vi "Image roto-translation top level.vi"(0 "ROI to crop (pixels)":T7={"Xmax"=2147483647, "Ymax"=2147483647, "Xmin"=0, "Ymin"=0}, 1 "Theta range (deg)":T6={"theta max (deg)"=180.0, "theta min (deg)"=-180.0}, 2 "Txy range (pixels)":T3={"Tx max (pix)"=2147483647, "Tx min (pix)"=-2147483648, "Ty max (pix)"=2147483647, "Ty min (pix)"=-2147483648}, 3 "Convergence tolerances":T4={"Tx,y tol (abs pix)"=0.001, "Rotation tol (abs deg)"=0.001, "Scale tol (rel fact)"=0.001}, 4 "Max. iters":i32=20, 5 "Controls":T2={"Auto ROI (for rot.)"=FALSE, "Apply scaling"=FALSE, "Apply rotation"=TRUE, "Apply Tx"=TRUE, "Apply Ty"=TRUE, "Keep proc. img"=FALSE}, 6 "Test image file path":path, 7 "R_min":dbl=150.0, 8 "Reference image file path":path, 9 "Pre-scale iters":i32=2) -> (12 "Iter":i32, 13 "Converged":bool, 14 "Scale factor":dbl, 15 "Rotation (deg)":dbl, 16 "Tx (pixels)":dbl, 17 "Ty (pixels)":dbl, 18 "Processed test img path":path, 19 "Error Out":errorcluster)   [LabVIEW 2022 SP3]
uses:
  Typedefs/ROI bounds.ctl
  Typedefs/Theta range.ctl
  Typedefs/Txy range.ctl
  Typedefs/Top level controls.ctl
  <vilib>/vision/NI_Vision_Development_Module.lvlib
panel:
  in  "ROI Color":u32(colorbox)=16711935
  out "Test image overlayed onto reference image (blend)":T1(plugin-control)
  out "Test image transformed":T1(plugin-control)
  out "Test image":T1(plugin-control)
  out "Convergence":T5(graph)
  out "Reference image":T1(plugin-control)
  # "ROI and Txy (pixels) are in image array coordinates. Origin is at top left, so positive y is towards the bottom of the image. positive x is towards the right of the image."
  # "Reference image info"
  # "Transformations are of test image relative to reference image, in image array coordinates"
  # "Paul Nathan 10/06/2015, \n07/12/2015, 22/03/2016, 06/04/2016, 19/04/2016, 23/06/2016"
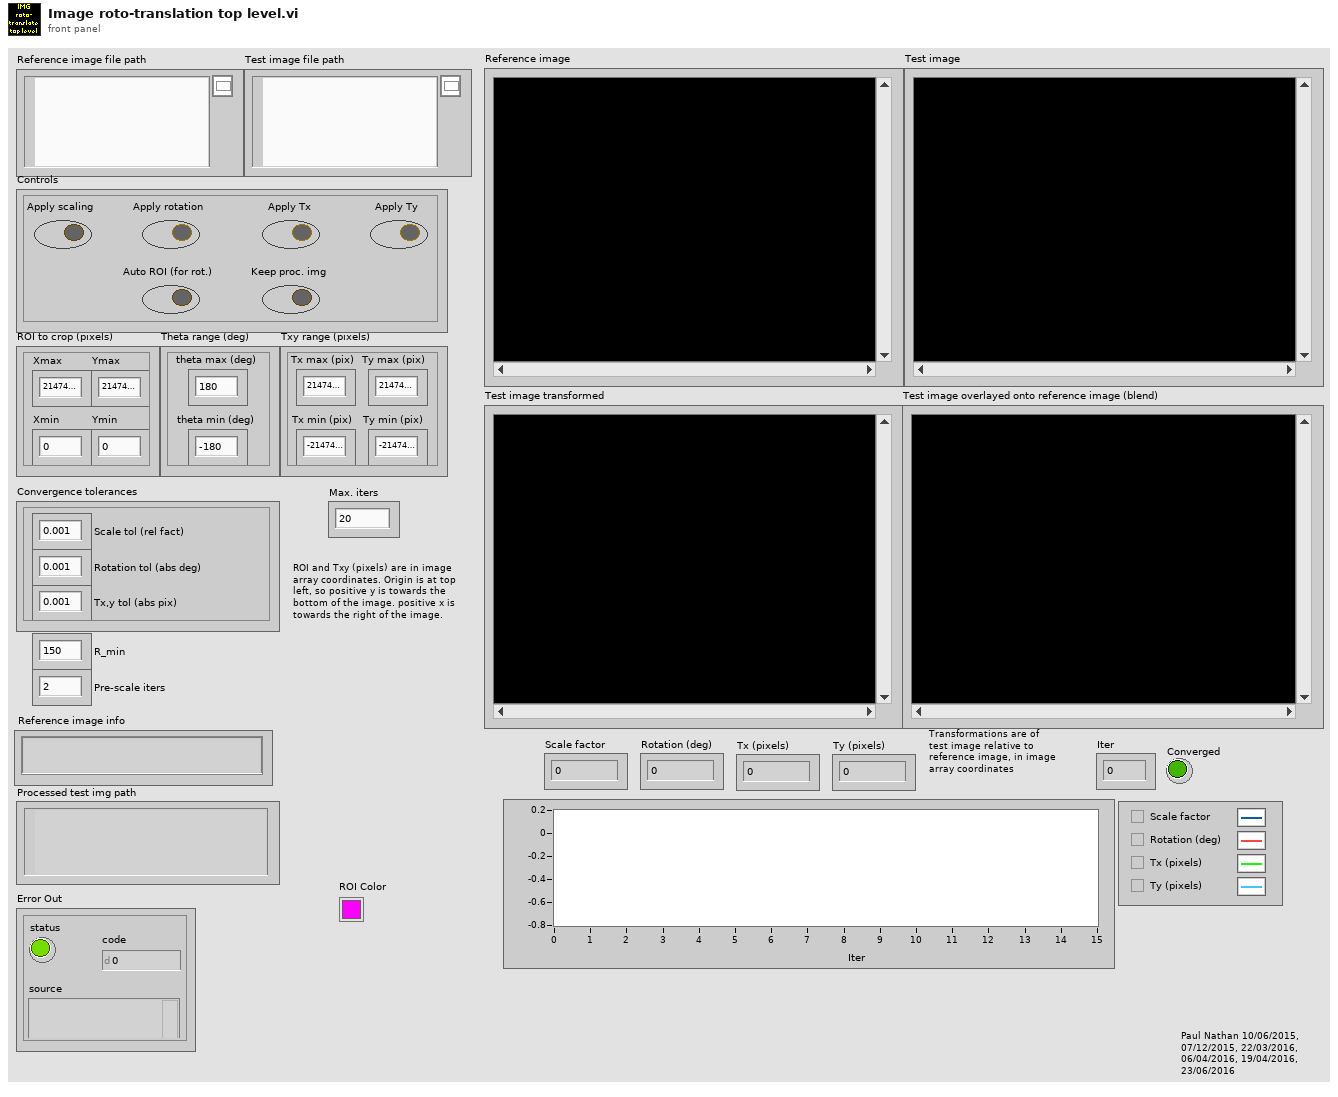
[diagram p1: front panel]
types:
  T1 = typedef "IMAQ Image.ctl" = refnum<image>
  T2 = typedef "Top level controls.ctl" = cluster{"Auto ROI (for rot.)":bool, "Apply scaling":bool, "Apply rotation":bool, "Apply Tx":bool, "Apply Ty":bool, "Keep proc. img":bool}
  T3 = typedef "Txy range.ctl" = cluster{"Tx max (pix)":i32, "Tx min (pix)":i32, "Ty max (pix)":i32, "Ty min (pix)":i32}
  T4 = cluster{"Tx,y tol (abs pix)":dbl, "Rotation tol (abs deg)":dbl, "Scale tol (rel fact)":dbl}
  T5 = cluster{dbl, dbl, "dx (pix)":dbl, "dy (pix)":dbl}
  T6 = typedef "Theta range.ctl" = cluster{"theta max (deg)":dbl, "theta min (deg)":dbl}
  T7 = typedef "ROI bounds.ctl" = cluster{"Xmax":i32, "Ymax":i32, "Xmin":i32, "Ymin":i32}
  T8 = cluster{dbl, dbl, "dx (pix)":dbl, "dy (pix)":dbl}[]
  T9 = typedef "Image Type" = u32
  T10 = cluster{"Xmin":i32, "Ymin":i32, "Xmax":i32, "Ymax":i32}
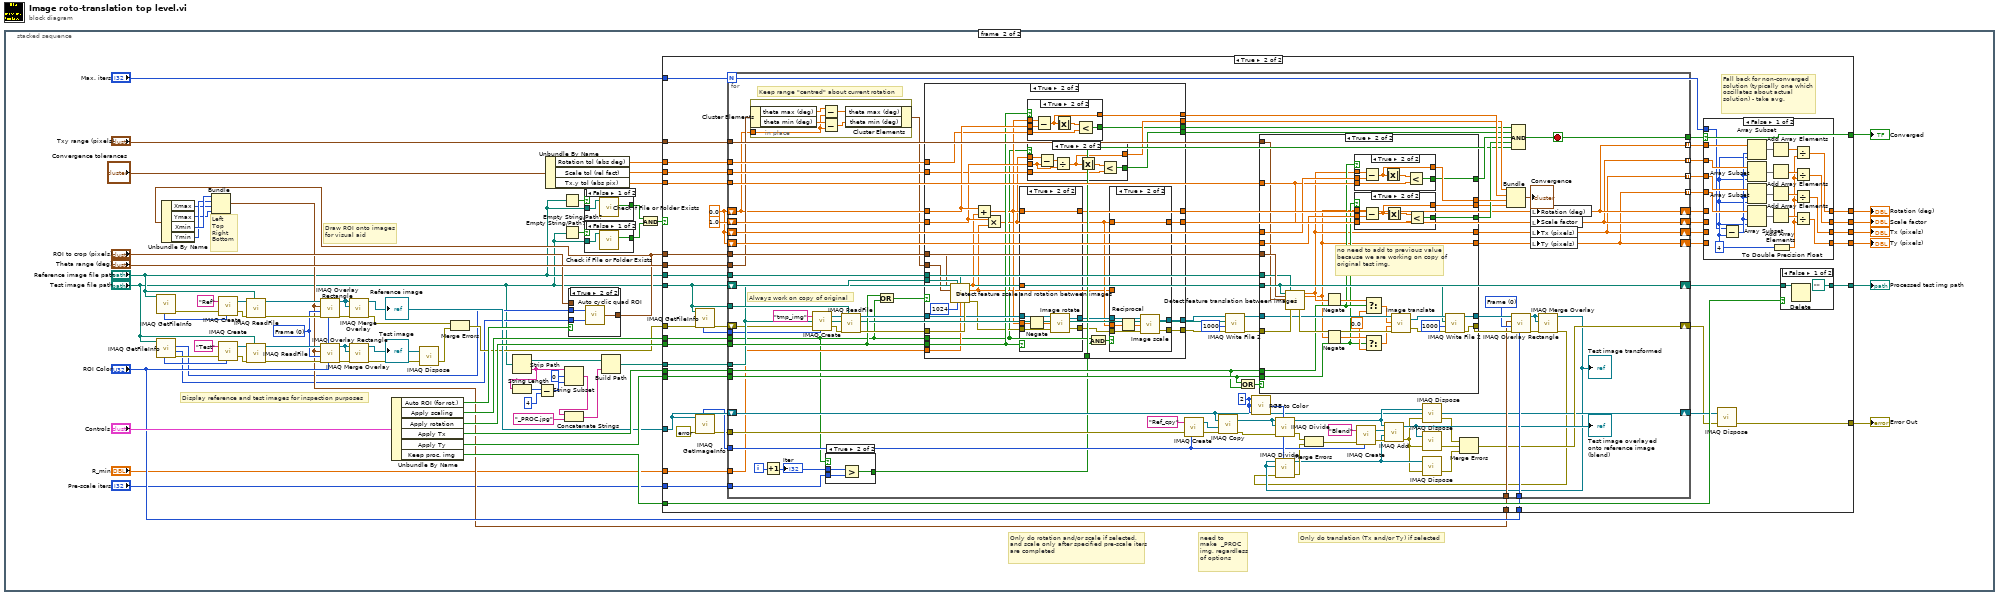
[diagram p0: block diagram]
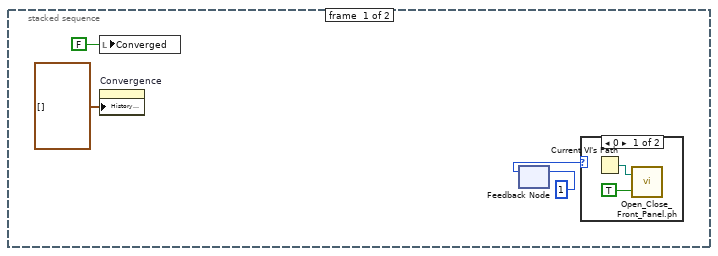
[diagram p2: hidden frame]
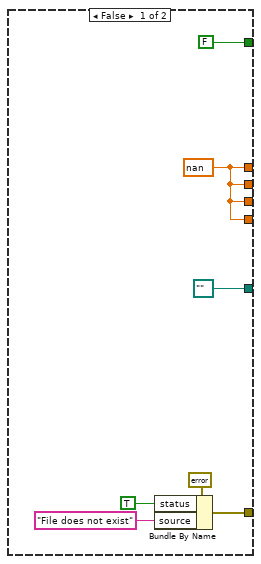
[diagram p4: hidden frame]
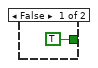
[diagram p5: hidden frame]
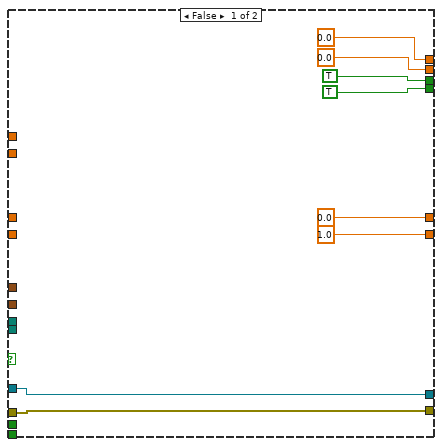
[diagram p6: hidden frame]
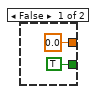
[diagram p7: hidden frame]
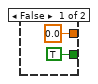
[diagram p8: hidden frame]
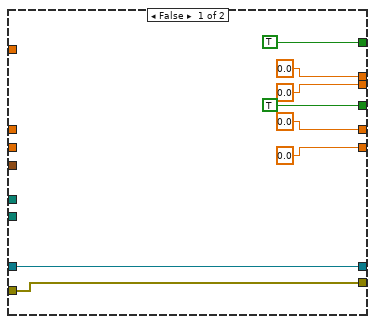
[diagram p11: hidden frame]
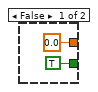
[diagram p12: hidden frame]
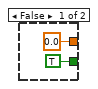
[diagram p13: hidden frame]
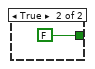
[diagram p16: hidden frame]
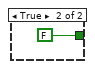
[diagram p17: hidden frame]
diagram:
  n1 = stacked-sequence {
    frame #0 {
      n2 = local write "Converged"(FALSE ("Converged")) -> ()
      n3 = property on="Convergence" class="WFChart (strict)"("History Data"=T8 []) -> ()  [unwired: 2 in, 2 out]
      n4 = feedback #1() -> (w2:i32)  [unwired: 1 in]
      n5 = feedback-in #1(1) -> ()
      n6 = case shown="0" w2 {
        frame 0 {
          n7 = Current VI's Path() -> (path=w5:path)
          n8 = call "Open_Close_Front_Panel.ph.vi"("openWindow (T)"=TRUE ("Front Panel Window:Open"), "VI path"=w5) -> ()  [unwired: 1 in, 1 out]
        }
        frame Default {
        }
      }
    }
    frame #1 {
      w29 = u32 0 items=["Frame", "Fill", "Highlight"] ("Drawing Mode (Frame)")
      # "Draw ROI onto images for visual aid"
      # "Display reference and test images for inspection purposes"
      # "Left\nTop\nRight\nBottom"
      # "Only do translation (Tx and/or Ty) if selected"
      # "Only do rotation and/or scale if selected,\nand scale only after specified pre-scale iters are completed"
      # "need to make  _PROC img, regardless of options"
      n9 = call "IMAQ GetFileInfo"("File Path"="Reference image file path") -> ("error out"=w45:errorcluster, "Image Type"=w44:T9)  [unwired: 4 in, 5 out]
      n10 = call "IMAQ GetFileInfo"("File Path"="Test image file path") -> ("error out"=w42:errorcluster, "Y Resolution"=w17:i32, "X Resolution"=w18:i32, "Image Type"=w43:T9)  [unwired: 4 in, 3 out]
      n11 = call "IMAQ Create"("Image Name"="Ref", "Image Type"=w44, "error in (no error)"=w45) -> ("New Image"=w47:T1, "error out"=w46:errorcluster)  [unwired: 2 in]
      n12 = call "IMAQ Create"("Image Name"="Test", "Image Type"=w43, "error in (no error)"=w42) -> ("New Image"=w40:T1, "error out"=w41:errorcluster)  [unwired: 2 in]
      n13 = call "IMAQ ReadFile"("File Path"="Reference image file path", "error in (no error)"=w46, "Image"=w47) -> ("error out"=w37:errorcluster, "Image Out"=w38:T1)  [unwired: 4 in, 3 out]
      n14 = call "IMAQ ReadFile"("File Path"="Test image file path", "error in (no error)"=w41, "Image"=w40) -> ("error out"=w30:errorcluster, "Image Out"=w31:T1)  [unwired: 4 in, 3 out]
      n15 = Unbundle By Name("Controls") -> ("Auto ROI (for rot.)"=w52:bool, "Apply scaling"=w51:bool, "Apply rotation"=w53:bool, "Apply Tx"=w54:bool, "Apply Ty"=w55:bool, "Keep proc. img"=w56:bool)
      n16 = Strip Path(path="Test image file path") -> (stripped path=w73:path, name=w79:string)
      n17 = String Length(string=w79) -> (length=w78:i32)
      n18 = Subtract(x=w78, y=4) -> (x-y=w72:i32)
      n19 = Unbundle By Name("Convergence tolerances") -> ("Rotation tol (abs deg)"=w60:dbl, "Scale tol (rel fact)"=w59:dbl, "Tx,y tol (abs pix)"=w58:dbl)
      n20 = Empty String/Path?(string/path="Reference image file path") -> (empty?=w10:bool)
      n21 = Empty String/Path?(string/path="Test image file path") -> (empty?=w8:bool)
      n22 = String Subset(string=w79, offset (0)=0, length (rest)=w72) -> (substring=w76:string)
      n23 = Concatenate Strings(w76, "_PROC.jpg" ("name or relative path")) -> (w74:string)
      n24 = case shown="True" w52 {
        tunnel: [w390 w391] -> w11
        tunnel: w18 -> [_ w393]
        tunnel: w17 -> [_ w392]
        tunnel: "ROI to crop (pixels)" -> [w390 _]
        frame False {
        }
        frame True {
          n25 = call "Auto cyclic quad ROI.vi"("img_H"=w392, "img_W"=w393) -> ("ROI to crop (pixels)"=w391:T7)
        }
      }
      n26 = Unbundle By Name(w11) -> ("Xmax"=w33:i32, "Ymax"=w32:i32, "Xmin"=w35:i32, "Ymin"=w34:i32)
      n27 = Bundle("Xmin"=w35, "Ymin"=w34, "Xmax"=w33, "Ymax"=w32) -> (w27:T10)  [unwired: 1 in]
      n28 = call "IMAQ Overlay Rectangle"("Color"="ROI Color", "error in (no error)"=w37, "Drawing Mode (Frame)"=w29, "Rectangle"=w27, "Image"=w38) -> ("error out"=w25:errorcluster, "Image Out"=w16:T1)  [unwired: 5 in]
      n29 = call "IMAQ Overlay Rectangle"("Color"="ROI Color", "error in (no error)"=w30, "Drawing Mode (Frame)"=w29, "Rectangle"=w27, "Image"=w31) -> ("error out"=w21:errorcluster, "Image Out"=w15:T1)  [unwired: 5 in]
      n30 = call "IMAQ Merge Overlay"("error in (no error)"=w25, "Image Dst"=w16, "Image Src"=w16) -> ("error out"=w24:errorcluster, "Image Dst Out"=w23:T1)  [unwired: 7 in]
      "Reference image" <- w23
      n31 = call "IMAQ Merge Overlay"("error in (no error)"=w21, "Image Dst"=w15, "Image Src"=w15) -> ("error out"=w20:errorcluster, "Image Dst Out"=w22:T1)  [unwired: 7 in]
      "Test image" <- w22
      n32 = call "IMAQ Dispose"("Image"=w22, "error in (no error)"=w20) -> ("error out"=w26:errorcluster)  [unwired: 4 in]
      n33 = Merge Errors(w24, w26) -> (w19:errorcluster)
      n34 = case shown="False" w10 {
        tunnel: [w388 FALSE ("file or folder exists?")] -> w67
        tunnel: "Reference image file path" -> [w387 _]
        frame False {
          n35 = call <vilib>:"Check if File or Folder Exists.vi"("path"=w387) -> ("file or folder exists?"=w388:bool)  [unwired: 8 in, 2 out]
        }
        frame True {
        }
      }
      n36 = case shown="False" w8 {
        tunnel: [w385 FALSE ("file or folder exists?")] -> w68
        tunnel: "Test image file path" -> [w384 _]
        frame False {
          n37 = call <vilib>:"Check if File or Folder Exists.vi"("path"=w384) -> ("file or folder exists?"=w385:bool)  [unwired: 8 in, 2 out]
        }
        frame True {
        }
      }
      n38 = Build Path(base path=w73, name or relative path=w74) -> (appended path=w80:path)
      n39 = And(x=w67, y=w68) -> (x .and. y?=w66:bool)
      n40 = case shown="True" w66 {
        tunnel: "Reference image file path" -> [_ w101]
        tunnel: "Max. iters" -> [_ w89]
        tunnel: w80 -> [_ w134]
        tunnel: [w86 w114] -> w63
        tunnel: [w86 w110] -> w64
        tunnel: "Test image file path" -> [_ w105]
        tunnel: [w86 w112] -> w62
        tunnel: w51 -> [_ w133]
        tunnel: w53 -> [_ w132]
        tunnel: w11 -> [_ w131]
        tunnel: w54 -> [_ w130]
        tunnel: w55 -> [_ w129]
        tunnel: "Theta range (deg)" -> [_ w128]
        tunnel: [path "" ("Test image file path") w125] -> w69
        tunnel: [w84 w96] -> w65
        tunnel: w56 -> [_ w127]
        tunnel: [w86 w108] -> w14
        tunnel: w60 -> [_ w122]
        tunnel: w59 -> [_ w121]
        tunnel: w58 -> [_ w120]
        tunnel: "Txy range (pixels)" -> [_ w119]
        tunnel: [FALSE w106] -> w49
        tunnel: w23 -> [_ w95]
        tunnel: w19 -> [_ w104]
        tunnel: "ROI Color" -> [_ w100]
        tunnel: w27 -> [_ w99]
        tunnel: "R_min" -> [_ w91]
        tunnel: "Pre-scale iters" -> [_ w90]
        frame False {
          w86 = nan ("Rotation (deg)")
          n41 = Bundle By Name(cluster=errorcluster {"status"=FALSE, "code"=0, "source"=""} ("error in (no error)"), "status"=TRUE, "source"="File does not exist") -> (w84:errorcluster)
        }
        frame True {
          w123 = 0.0 ("Rotation (deg)")
          # "Fall back for non-converged solution (typically one which oscillates about actual solution) - take avg."
          n42 = call "IMAQ GetImageInfo"("error in (no error)"=errorcluster {"status"=FALSE, "code"=0, "source"=""}, "Image"=w95) -> ("error out"=w92:errorcluster, "Image Type"=w94:T9)  [unwired: 2 in, 6 out]
          n43 = call "IMAQ GetFileInfo"("error in (no error)"=w104, "File Path"=w105) -> ("error out"=w103:errorcluster, "Image Type"=w102:T9)  [unwired: 3 in, 5 out]
          n44 = for {
            N: w89 -> [_]
            tunnel: w101 -> [w194]
            shift-right: [w190] -> w126
            shift-left: w105 -> [w219]
            tunnel: w134 -> [w190]
            shift-right: [w148] -> w97
            shift-left: w103 -> [w177]
            tunnel: w133 -> [w135]
            tunnel: w132 -> [w195]
            tunnel: w131 -> [w218]
            tunnel: w130 -> [w192]
            tunnel: w129 -> [w193]
            tunnel: w128 -> [w184]
            tunnel: w105 -> [w212]
            shift-right: [w181] -> w113
            shift-left: w123 -> [w183]
            shift-right: [w180] -> w111
            shift-left: 1.0 ("Rotation (deg)") -> [w205]
            shift-right: [w179] -> w109
            shift-left: w123 -> [w203]
            shift-right: [w142] -> w107
            shift-left: w123 -> [w202]
            tunnel: w122 -> [w208]
            tunnel: w121 -> [w197]
            tunnel: w120 -> [w196]
            tunnel: w119 -> [w185]
            tunnel: [w181] -> w118 mode=indexing
            tunnel: [w180] -> w117 mode=indexing
            tunnel: [w179] -> w116 mode=indexing
            tunnel: [w142] -> w115 mode=indexing
            tunnel: [w178] -> w106
            tunnel: w102 -> [w176]
            tunnel: w92 -> [w161]
            tunnel: w94 -> [w163]
            tunnel: w100 -> [w171]
            tunnel: w99 -> [w170]
            shift-right: [w147] -> w98
            shift-left: w95 -> [w147]
            tunnel: w91 -> [w140]
            tunnel: w90 -> [w137]
            i -> [w139]
            stop <- w178 stop-if-true
            w169 = u8 2 ("R")
            w172 = u32 0 items=["Frame", "Fill", "Highlight"] ("Drawing Mode (Frame)")
            # "Keep range \"centred\" about current rotation"
            # "Always work on copy of original"
            n45 = in-place {
              in-place-border: w183 -> [w226]
              n46 = in-place-cluster #2(w184) -> ("theta max (deg)"=w228:dbl, "theta min (deg)"=w227:dbl)
              n47 = Subtract(x=w228, y=w226) -> (x-y=w225:dbl)
              n48 = Subtract(x=w227, y=w226) -> (x-y=w224:dbl)
              n49 = in-place-cluster #2("theta max (deg)"=w225, "theta min (deg)"=w224) -> (w182:T6)
            }
            n50 = Increment(x=w139) -> (x+1=w138:i32)
            "Iter" <- w138
            n51 = call "IMAQ Create"("Image Name"="tmp_img", "Image Type"=w176, "error in (no error)"=w177) -> ("New Image"=w216:T1, "error out"=w217:errorcluster)  [unwired: 2 in]
            n52 = case shown="True" w135 {
              tunnel: w138 -> [_ w223]
              tunnel: w137 -> [_ w222]
              tunnel: [TRUE w221] -> w136
              frame False {
              }
              frame True {
                n53 = Greater?(x=w223, y=w222) -> (0:w221:bool)
              }
            }
            n54 = call "IMAQ ReadFile"("File Path"=w212, "error in (no error)"=w217, "Image"=w216) -> ("error out"=w214:errorcluster, "Image Out"=w213:T1)  [unwired: 4 in, 3 out]
            n55 = Or(x=w195, y=w135) -> (x .or. y?=w186:bool)
            n56 = case shown="True" w186 {
              tunnel: w219 -> [_ w267]
              tunnel: w218 -> [_ w266]
              tunnel: w182 -> [_ w265]
              tunnel: w214 -> [w229 w264]
              tunnel: w213 -> [w230 w263]
              tunnel: w183 -> [_ w262]
              tunnel: w208 -> [_ w261]
              tunnel: [0.0 w260] -> w207
              tunnel: [0.0 w259] -> w206
              tunnel: w205 -> [_ w258]
              tunnel: [TRUE w257] -> w201
              tunnel: [TRUE w256] -> w200
              tunnel: w197 -> [_ w255]
              tunnel: [1.0 w243] -> w180
              tunnel: [0.0 w246] -> w181
              tunnel: w135 -> [_ w240]
              tunnel: w195 -> [_ w254]
              tunnel: w194 -> [_ w253]
              tunnel: [w229 w249] -> w188
              tunnel: [w230 w248] -> w187
              tunnel: w140 -> [_ w241]
              tunnel: w136 -> [_ w238]
              frame False {
              }
              frame True {
                n57 = call "Detect feature scale and rotation between images.vi"("ROI to crop (pixels)"=w266, "Test image file path"=w267, "Reference image file path"=w253, "Theta range (deg)"=w265, "Log-polar transform size"=1024, "R_min"=w241, "Error In"=w264) -> ("Rotation (deg)"=w245:dbl, "Scale factor"=w242:dbl, "Error out"=w252:errorcluster)  [unwired: 4 in, 2 out]
                n58 = Add(x=w262, y=w245) -> (x+y=w247:dbl)
                n59 = Multiply(x=w258, y=w242) -> (x*y=w244:dbl)
                n60 = case shown="True" w254 {
                  tunnel: w263 -> [w287 w290]
                  tunnel: w252 -> [w286 w294]
                  tunnel: w247 -> [_ w291]
                  tunnel: [w287 w293] -> w251
                  tunnel: [w286 w292] -> w250
                  tunnel: w247 -> [_ w288]
                  tunnel: [w285 w288] -> w246
                  tunnel: w245 -> [w285 _]
                  frame False {
                  }
                  frame True {
                    n61 = Negate(x=w291) -> (-x=w289:dbl)
                    n62 = call "Image rotate.vi"("Error in"=w294, "Rotation angle, ccw+ (deg)"=w289, "Image in"=w290) -> ("Error Out"=w292:errorcluster, "Image Out"=w293:T1)
                  }
                }
                n63 = case shown="True" w254 {
                  tunnel: w262 -> [_ w284]
                  tunnel: w261 -> [_ w283]
                  tunnel: [0.0 w281] -> w260
                  tunnel: [TRUE w280] -> w257
                  tunnel: w247 -> [_ w279]
                  frame False {
                  }
                  frame True {
                    n64 = Subtract(x=w279, y=w284) -> (x-y=w281:dbl)
                    n65 = Absolute Value(x=w281) -> (abs(x)=w282:dbl)
                    n66 = Less?(x=w282, y=w283) -> (x < y?=w280:bool)
                  }
                }
                n67 = case shown="True" w240 {
                  tunnel: [0.0 w275] -> w259
                  tunnel: w258 -> [_ w273]
                  tunnel: [TRUE w272] -> w256
                  tunnel: w255 -> [_ w271]
                  tunnel: w244 -> [_ w270]
                  frame False {
                  }
                  frame True {
                    n68 = Subtract(x=w270, y=w273) -> (x-y=w276:dbl)
                    n69 = Divide(x=w276, y=w273) -> (x/y=w275:dbl)
                    n70 = Absolute Value(x=w275) -> (abs(x)=w274:dbl)
                    n71 = Less?(x=w274, y=w271) -> (x < y?=w272:bool)
                  }
                }
                n72 = And(x=w240, y=w238) -> (x .and. y?=w239:bool)
                n73 = case shown="True" w239 {
                  tunnel: w251 -> [w297 w304]
                  tunnel: [w297 w303] -> w248
                  tunnel: w250 -> [w296 w302]
                  tunnel: [w296 w301] -> w249
                  tunnel: w244 -> [_ w300]
                  tunnel: w244 -> [_ w298]
                  tunnel: [w295 w298] -> w243
                  tunnel: w242 -> [w295 _]
                  frame False {
                  }
                  frame True {
                    n74 = Reciprocal(x=w300) -> (1/x=w299:dbl)
                    n75 = call "Image scale.vi"("Error in"=w302, "Scale factor"=w299, "Image in"=w304) -> ("Error Out"=w301:errorcluster, "Image Out"=w303:T1)
                  }
                }
              }
            }
            n76 = call "IMAQ Create"("Image Name"="Ref_cpy", "Image Type"=w163, "error in (no error)"=w161) -> ("New Image"=w162:T1, "error out"=w160:errorcluster)  [unwired: 2 in]
            n77 = call "IMAQ Copy"("error in (no error)"=w160, "Image Dst"=w162, "Image Src"=w147) -> ("error out"=w152:errorcluster, "Image Dst Out"=w165:T1)  [unwired: 3 in]
            n78 = call-poly "IMAQ Write File 2"("error in (no error)"=w188, "Image Quality"=u32 1000, "File Path"=w190, "Image"=w187) -> ("error out"=w211:errorcluster, "Image Out (duplicate)"=w210:T1)  [unwired: 6 in]
            n79 = Or(x=w193, y=w192) -> (x .or. y?=w191:bool)
            n80 = call <vilib>:"RGB to Color.vi"("B"=w169, "G"=w169, "R"=w169) -> ("Color"=w168:u32)
            n81 = case shown="True" w191 {
              tunnel: w218 -> [_ w335]
              tunnel: [w305 w334] -> w173
              tunnel: w211 -> [w305 w332]
              tunnel: w210 -> [w306 w331]
              tunnel: [w306 w330] -> w174
              tunnel: [0.0 w329] -> w204
              tunnel: [0.0 w328] -> w141
              tunnel: w203 -> [_ w327]
              tunnel: w202 -> [_ w326]
              tunnel: w192 -> [_ w318]
              tunnel: w193 -> [_ w317]
              tunnel: [TRUE ("f") w319] -> w199
              tunnel: [TRUE ("f") w316] -> w198
              tunnel: w196 -> [_ w325]
              tunnel: [0.0 ("dy (pix)") w314] -> w142
              tunnel: [0.0 ("dx (pix)") w315] -> w179
              tunnel: w194 -> [_ w324]
              tunnel: w190 -> [_ w323]
              tunnel: w185 -> [_ w313]
              frame False {
              }
              frame True {
                w320 = 0.0 ("f")
                # "no need to add to previous value because we are working on copy of original test img."
                n82 = call "Detect feature translation between images.vi"("Test image file path"=w323, "ROI to crop (pixels)"=w335, "Txy range (pixels)"=w313, "Reference image file path"=w324, "Error In"=w332) -> ("Error out"=w333:errorcluster, "dx (pix)"=w315:dbl, "dy (pix)"=w314:dbl)  [unwired: 10 in, 2 out]
                n83 = Negate(x=w315) -> (-x=w337:dbl)
                n84 = Negate(x=w314) -> (-x=w336:dbl)
                n85 = case shown="True" w318 {
                  tunnel: [0.0 w356] -> w329
                  tunnel: w327 -> [_ w354]
                  tunnel: w325 -> [_ w353]
                  tunnel: w315 -> [_ w352]
                  tunnel: [TRUE w351] -> w319
                  frame False {
                  }
                  frame True {
                    n86 = Subtract(x=w352, y=w354) -> (x-y=w356:dbl)
                    n87 = Absolute Value(x=w356) -> (abs(x)=w355:dbl)
                    n88 = Less?(x=w355, y=w353) -> (x < y?=w351:bool)
                  }
                }
                n89 = case shown="True" w317 {
                  tunnel: [0.0 w348] -> w328
                  tunnel: w326 -> [_ w346]
                  tunnel: w325 -> [_ w345]
                  tunnel: w314 -> [_ w344]
                  tunnel: [TRUE w343] -> w316
                  frame False {
                  }
                  frame True {
                    n90 = Subtract(x=w344, y=w346) -> (x-y=w348:dbl)
                    n91 = Absolute Value(x=w348) -> (abs(x)=w347:dbl)
                    n92 = Less?(x=w347, y=w345) -> (x < y?=w343:bool)
                  }
                }
                n93 = Select(t=w337, s=w318, f=w320) -> (s? t:f=w322:dbl)
                n94 = Select(t=w336, s=w317, f=w320) -> (s? t:f=w321:dbl)
                n95 = call "Image translate.vi"("Error in"=w333, "Ty (pix)"=w321, "Tx (pix)"=w322, "Image in"=w331) -> ("Error Out"=w338:errorcluster, "Image Out"=w339:T1)
                n96 = call-poly "IMAQ Write File 2"("error in (no error)"=w338, "Image Quality"=u32 1000, "File Path"=w323, "Image"=w339) -> ("error out"=w334:errorcluster, "Image Out (duplicate)"=w330:T1)  [unwired: 6 in]
              }
            }
            n97 = call "IMAQ Divide"("Image Src A"=w165, "Constant"=w168, "Image Dst"=w165, "error in (no error)"=w152) -> ("Image Dst Out"=w153:T1, "error out"=w159:errorcluster)  [unwired: 3 in]
            n98 = Bundle(w206, w207, w204, w141) -> (→"Convergence":cluster{dbl, dbl, dbl, dbl})  [unwired: 1 in]
            n99 = Compound Arithmetic op=AND(w201, w200, w199, w198, w136) -> (w178:bool)
            n100 = call "IMAQ Overlay Rectangle"("Color"=w171, "error in (no error)"=w173, "Drawing Mode (Frame)"=w172, "Rectangle"=w170, "Image"=w174) -> ("error out"=w146:errorcluster, "Image Out"=w143:T1)  [unwired: 5 in]
            n101 = local write "Rotation (deg)"(w181) -> ()
            n102 = local write "Scale factor"(w180) -> ()
            n103 = local write "Tx (pixels)"(w179) -> ()
            n104 = local write "Ty (pixels)"(w142) -> ()
            n105 = call "IMAQ Merge Overlay"("error in (no error)"=w146, "Image Dst"=w143, "Image Src"=w143) -> ("error out"=w144:errorcluster, "Image Dst Out"=w145:T1)  [unwired: 7 in]
            "Test image transformed" <- w145
            n106 = call "IMAQ Divide"("Image Src A"=w145, "Constant"=w168, "Image Dst"=w145, "error in (no error)"=w144) -> ("Image Dst Out"=w155:T1, "error out"=w158:errorcluster)  [unwired: 3 in]
            n107 = Merge Errors(w159, w158) -> (w157:errorcluster)
            n108 = call "IMAQ Create"("Image Name"="Blend", "Image Type"=w163, "error in (no error)"=w157) -> ("New Image"=w167:T1, "error out"=w166:errorcluster)  [unwired: 2 in]
            n109 = call "IMAQ Add"("Image Src A"=w153, "Image Dst"=w167, "Image Src B"=w155, "error in (no error)"=w166) -> ("Image Dst Out"=w156:T1, "error out"=w154:errorcluster)  [unwired: 3 in]
            "Test image overlayed onto reference image (blend)" <- w156
            n110 = call "IMAQ Dispose"("Image"=w153, "error in (no error)"=w154) -> ("error out"=w151:errorcluster)  [unwired: 4 in]
            n111 = call "IMAQ Dispose"("Image"=w156, "error in (no error)"=w154) -> ("error out"=w150:errorcluster)  [unwired: 4 in]
            n112 = call "IMAQ Dispose"("Image"=w155, "error in (no error)"=w154) -> ("error out"=w149:errorcluster)  [unwired: 4 in]
            n113 = Merge Errors(w151, w150, w149) -> (w148:errorcluster)
          }
          n114 = case shown="False" w106 {
            tunnel: w118 -> [w376 _]
            tunnel: w117 -> [w365 _]
            tunnel: w116 -> [w364 _]
            tunnel: w115 -> [w363 _]
            tunnel: [w368 w380] -> w114
            tunnel: w113 -> [_ w380]
            tunnel: [w369 w379] -> w112
            tunnel: w111 -> [_ w379]
            tunnel: [w370 w378] -> w110
            tunnel: w109 -> [_ w378]
            tunnel: [w371 w377] -> w108
            tunnel: w107 -> [_ w377]
            tunnel: w89 -> [w357 _]
            frame False {
              w358 = 4 ("number")
              n115 = Subtract(x=w357, y=w358) -> (x-y=w359:i32)
              n116 = Array Subset(array=w376, index=w359, length=w358) -> (w366:dbl[])
              n117 = Array Subset(array=w365, index=w359, length=w358) -> (w362:dbl[])
              n118 = Array Subset(array=w364, index=w359, length=w358) -> (w361:dbl[])
              n119 = Array Subset(array=w363, index=w359, length=w358) -> (w360:dbl[])
              n120 = Add Array Elements(numeric array=w366) -> (sum=w375:dbl)
              n121 = Add Array Elements(numeric array=w362) -> (sum=w374:dbl)
              n122 = Add Array Elements(numeric array=w361) -> (sum=w373:dbl)
              n123 = Add Array Elements(numeric array=w360) -> (sum=w372:dbl)
              n124 = To Double Precision Float(number=w358) -> (double precision float=w367:dbl)
              n125 = Divide(x=w375, y=w367) -> (x/y=w368:dbl)
              n126 = Divide(x=w374, y=w367) -> (x/y=w369:dbl)
              n127 = Divide(x=w373, y=w367) -> (x/y=w370:dbl)
              n128 = Divide(x=w372, y=w367) -> (x/y=w371:dbl)
            }
            frame True {
            }
          }
          n129 = call "IMAQ Dispose"("Image"=w98, "error in (no error)"=w97) -> ("error out"=w96:errorcluster)  [unwired: 4 in]
          n130 = case shown="False" w127 {
            tunnel: w126 -> [w381 w383]
            tunnel: [path "" ("Test image file path") w383] -> w125
            frame False {
              n131 = Delete(path (use dialog)=w381) -> ()  [unwired: 4 in, 3 out]
            }
            frame True {
            }
          }
        }
      }
      "Processed test img path" <- w69
      "Error Out" <- w65
      "Tx (pixels)" <- w64
      "Ty (pixels)" <- w14
      "Rotation (deg)" <- w63
      "Scale factor" <- w62
      "Converged" <- w49
    }
  }
